vi "UDP Multicast Sender.vi"(4 "Num Of Times To Send Message":u32, 5 "Data String":string="Sent over UDP Multicast", 6 "error in (no error)":errorcluster, 7 "Multicast Address":string="234.5.6.7", 8 "Remote Port":i32=3456, 9 "UDP Network Connection Refnum":refnum<k16>) -> ()   [LabVIEW 2012]
doc: "UDP multicast will allow LabVIEW to send data to a multicast group or to receive data sent to a multicast group. In LabVIEW, UDP multicast is used in very much the same way as UDP. The main difference is there are two new parameters, TTL and Multicast Address, on the UDP Multicast Open. \n\nWhen sending to a multicast group the default time-to-live (TTL) is 1, which only allows the packet to go to the local subnet. When a router receives a multicast packet, it decrements the packets TTL, and if the TTL is greater than 0, forwards the packet to other routers.\nA multicast group is defined by having a multicast IP address in the range 224.0.0.0-239.255.255.255."
panel:
  out "error out":errorcluster
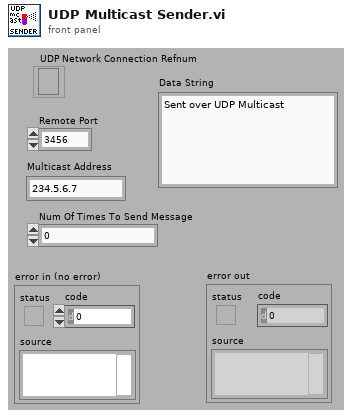
[diagram p1: front panel]
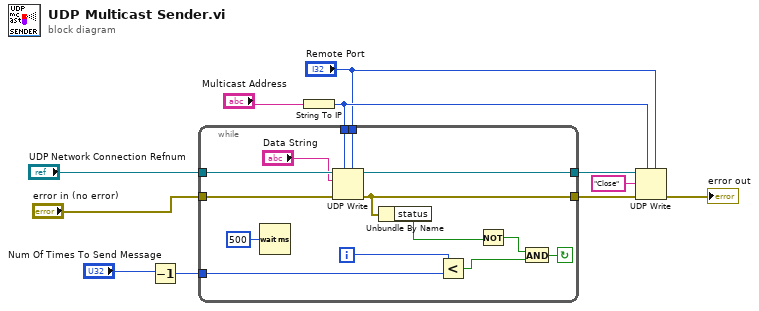
[diagram p0: block diagram]
diagram:
  n1 = Decrement(x="Num Of Times To Send Message") -> (x-1=w2:u32)
  n2 = String To IP(1:"Multicast Address") -> (0:w8:u32)
  n3 = while {
    tunnel: "UDP Network Connection Refnum" -> [w25]
    tunnel: "error in (no error)" -> [w24]
    tunnel: [w17] -> w5
    tunnel: "Remote Port" -> [w23]
    tunnel: w8 -> [w22]
    tunnel: [w15] -> w6
    tunnel: w2 -> [w12]
    i -> [w14]
    stop <- w18 continue-if-true
    n4 = Wait (ms)(milliseconds to wait=u32 500) -> ()  [unwired: 1 out]
    n5 = UDP Write(address=w22, port or service name=w23, connection ID=w25, data in="Data String", 8:w24) -> (error out=w17:errorcluster, 3:w15:refnum<k16>)  [unwired: 1 out]
    n6 = Unbundle By Name(w17) -> ("status"=w19:bool)
    n7 = Less?(x=w14, y=w12) -> (x < y?=w13:bool)
    n8 = Not(x=w19) -> (.not. x?=w16:bool)
    n9 = And(x=w16, y=w13) -> (x .and. y?=w18:bool)
  }
  n10 = UDP Write(address=w8, port or service name="Remote Port", connection ID=w6, data in="Close", 8:w5) -> (error out=→"error out":errorcluster)  [unwired: 2 out]
